vi "Monitor Loop Rate - Latching.vi"(9 "Reset":bool, 10 "Count(Ticks)":u32) -> (0 "Actual Loop Rate (Ticks)":u32, 1 "Late? (Latched)":bool, 2 "Tick Count (Ticks)":u32)   [LabVIEW 2014, in "SYSID.lvlib"]
doc: "This VI will monitor the rate of a loop on FPGA. It calculates the number of ticks that have passed since the last call and compares it with the desired count. If more ticks have passed than desired, the Late? Boolean latches to TRUE until reset.\n\n<B>Inputs:</B>\n<B>Count(Ticks)</B> - The desired number of ticks since the last call.\n<B>Reset</B> - Resets the Late? Boolean.\n\n<B>Outputs:</B>\n<B>Tick Count (Ticks)</B> - Returns the value of the free running tick counter.\n<B>Late? (Latched)</B> - Indicates if more FPGA Ticks have passed than the specified number. This Boolean value is latched until reset.\n<B>Actual Loop Rate (Ticks)</B> - The number of ticks that have passed since the last call."
uses:
  SYSID.lvlib
  <vilib>/rvi/Emulation/niFpgaProcessEmulError.vi
  Instance           2 36Saved   Monitor Loop Rate - Latching .vi
  <vilib>/rvi/Emulation/niFpgaSctlEmulationGetInTimedLoop.vi
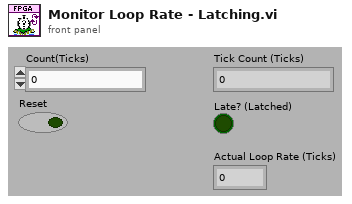
[diagram p1: front panel]
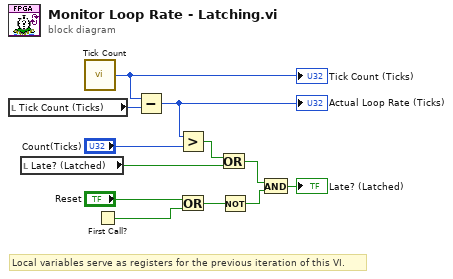
[diagram p0: block diagram]
diagram:
  # "Local variables serve as registers for the previous iteration of this VI."
  n1 = local read "Tick Count (Ticks)"() -> (w11:u32)
  n2 = local read "Late? (Latched)"() -> (w9:bool)
  n3 = call "Tick Count"() -> ("Tick Count(Ticks)"=w12:u32)
  "Tick Count (Ticks)" <- w12
  n4 = First Call?() -> (First Call?: T/F=w7:bool)
  n5 = Subtract(x=w12, y=w11) -> (x-y=w1:u32)
  "Actual Loop Rate (Ticks)" <- w1
  n6 = Greater?(x=w1, y="Count(Ticks)") -> (0:w10:bool)
  n7 = Or(x="Reset", y=w7) -> (x .or. y?=w6:bool)
  n8 = Or(x=w10, y=w9) -> (x .or. y?=w4:bool)
  n9 = Not(x=w6) -> (.not. x?=w3:bool)
  n10 = And(x=w4, y=w3) -> (x .and. y?=→"Late? (Latched)":bool)
